vi "Error Query.vi"(0 "VISA resource name":refnum<visa-resource-name>, 11 "error in (no error)":errorcluster) -> (4 "VISA resource name out":refnum<visa-resource-name>, 8 "Error":i32, 10 "Error Message":string, 15 "error out":errorcluster)   [LabVIEW 2019, in "Lake Shore Cryotronics 340.lvlib"]
doc: "This VI reads an error from the instrument. This instrument does not support an error query and this VI returns a warning code if it is executed."
uses:
  Lake Shore Cryotronics 340.lvlib
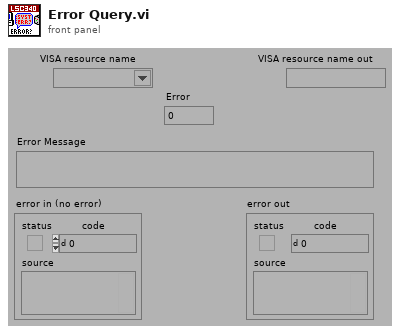
[diagram p1: front panel]
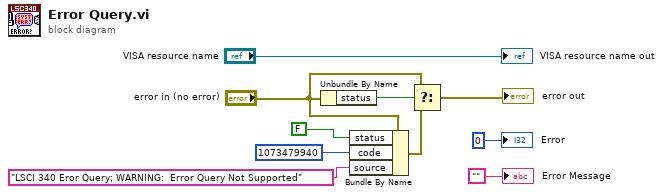
[diagram p0: block diagram]
diagram:
  n1 = Unbundle By Name("error in (no error)") -> ("status"=w2:bool)
  n2 = Bundle By Name(cluster="error in (no error)", "status"=FALSE, "code"=1073479940, "source"="LSCI 340 Eror Query; WARNING:  Error Query Not Supported") -> (w1:errorcluster)
  n3 = Select(t="error in (no error)", s=w2, f=w1) -> (s? t:f=→"error out":errorcluster)
  "Error Message" <- ""
  "Error" <- 0
  "VISA resource name out" <- "VISA resource name"
